vi "Icon Resolve Color.vi"(10 "color":u32(colorbox), 11 "8-bit colors":u32[](array[colorbox])) -> (2 "8-bit color":u32(colorbox), 3 "index":i32)   [LabVIEW 2019, in "Builtins.lvlib"]
doc: "Resolves the color to the nearest <b>8-bit colors</b> array.\n\nCreated by: Ryan Pacini"
uses:
  Builtins.lvlib
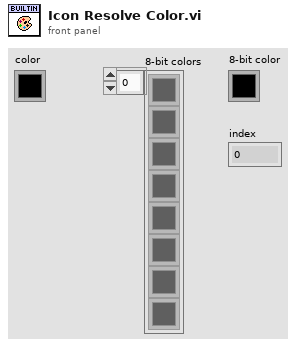
[diagram p1: front panel]
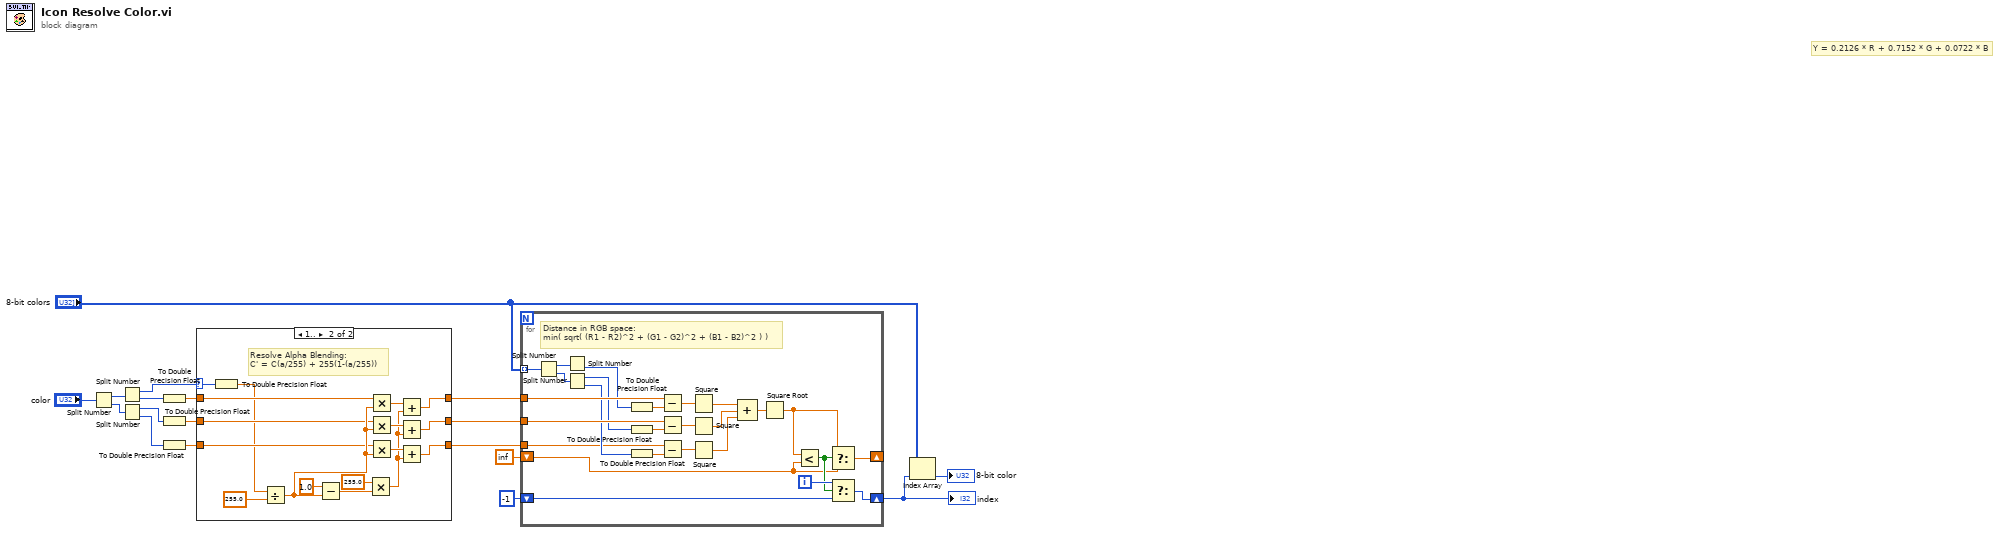
[diagram p0: block diagram]
diagram:
  # "Y = 0.2126 * R + 0.7152 * G + 0.0722 * B"
  n1 = Split Number(x="color") -> (hi(x)=w15:u16, lo(x)=w16:u16)
  n2 = Split Number(x=w15) -> (hi(x)=w3:u8, lo(x)=w14:u8)
  n3 = Split Number(x=w16) -> (hi(x)=w13:u8, lo(x)=w12:u8)
  n4 = To Double Precision Float(number=w14) -> (double precision float=w11:dbl)
  n5 = To Double Precision Float(number=w13) -> (double precision float=w10:dbl)
  n6 = To Double Precision Float(number=w12) -> (double precision float=w9:dbl)
  n7 = case shown="1.." w3 {
    selector: w3 -> [_ w23]
    tunnel: w11 -> [w21 w29]
    tunnel: w10 -> [w20 w28]
    tunnel: w9 -> [w19 w27]
    tunnel: [w21 w26] -> w7
    tunnel: [w20 w25] -> w6
    tunnel: [w19 w24] -> w5
    frame 0 {
    }
    frame 1.. {
      # "Resolve Alpha Blending:\nC' = C(a/255) + 255(1-(a/255))"
      n8 = To Double Precision Float(number=w23) -> (double precision float=w22:dbl)
      n9 = Divide(x=w22, y=255.0) -> (x/y=w31:dbl)
      n10 = Subtract(x=1.0, y=w31) -> (x-y=w35:dbl)
      n11 = Multiply(x=255.0, y=w35) -> (x*y=w30:dbl)
      n12 = Multiply(x=w29, y=w31) -> (x*y=w34:dbl)
      n13 = Multiply(x=w28, y=w31) -> (x*y=w33:dbl)
      n14 = Multiply(x=w27, y=w31) -> (x*y=w32:dbl)
      n15 = Add(x=w34, y=w30) -> (x+y=w26:dbl)
      n16 = Add(x=w33, y=w30) -> (x+y=w25:dbl)
      n17 = Add(x=w32, y=w30) -> (x+y=w24:dbl)
    }
  }
  n18 = for {
    tunnel: w7 -> [w62]
    tunnel: w6 -> [w60]
    tunnel: w5 -> [w57]
    tunnel: "8-bit colors" -> [w46] mode=indexing
    shift-right: [w42] -> w18
    shift-left: -1 -> [w41]
    shift-right: [w40] -> _
    shift-left: inf ("double precision float") -> [w39]
    i -> [w44]
    # "Distance in RGB space:\nmin( sqrt( (R1 - R2)^2 + (G1 - G2)^2 + (B1 - B2)^2 ) )"
    n19 = Split Number(x=w46) -> (hi(x)=w64:u16, lo(x)=w63:u16)
    n20 = Split Number(x=w64) -> (lo(x)=w61:u8)  [unwired: 1 out]
    n21 = Split Number(x=w63) -> (hi(x)=w59:u8, lo(x)=w58:u8)
    n22 = To Double Precision Float(number=w61) -> (double precision float=w49:dbl)
    n23 = To Double Precision Float(number=w59) -> (double precision float=w48:dbl)
    n24 = To Double Precision Float(number=w58) -> (double precision float=w47:dbl)
    n25 = Subtract(x=w62, y=w49) -> (x-y=w56:dbl)
    n26 = Subtract(x=w60, y=w48) -> (x-y=w55:dbl)
    n27 = Subtract(x=w57, y=w47) -> (x-y=w54:dbl)
    n28 = Square(x=w56) -> (x^2=w53:dbl)
    n29 = Square(x=w55) -> (x^2=w52:dbl)
    n30 = Square(x=w54) -> (x^2=w51:dbl)
    n31 = Compound Arithmetic op=ADD(w53, w52, w51) -> (w50:dbl)
    n32 = Square Root(x=w50) -> (sqrt(x)=w45:dbl)
    n33 = Less?(x=w45, y=w39) -> (x < y?=w43:bool)
    n34 = Select(t=w45, s=w43, f=w39) -> (s? t:f=w40:dbl)
    n35 = Select(t=w44, s=w43, f=w41) -> (s? t:f=w42:i32)
  }
  "index" <- w18
  n36 = Index Array(array="8-bit colors", index=w18) -> (element=→"8-bit color":u32)
